vi "Broadcast Sonicator Settings.vi"(8 "error in (no error)":errorcluster, 10 "Message Queues":T5, 11 "Scale Module Config":T1={"GUID"="", "Drop Coords"={"Horizontal"=0, "Vertical"=0}, "Process Name"="", "Queue Name"="", "Settings"={"Cycle Period"=500.0, "Mettler"={"VISA resource name"="", "Simulated?"=FALSE}, "Scale Type"=""}, "Load Count"=0}) -> (0 "error out":errorcluster)   [LabVIEW 2018, in "Sonicator Module.lvlib"]
uses:
  Sonicator Module.lvlib
  Sonicator Message Queues.ctl
  support/Message Queue/Message Cluster.ctl
  Controls/Sonicator Module Config Cluster.ctl
  <vilib>/Utility/miscctls.llb/LVPoint32TypeDef.ctl
  Controls/Sonicator Module Settings Cluster.ctl
  Mettler Toledo/Controls/Settings Cluster.ctl
  support/Message Queue/Enqueue Message (Single).vi
  support/Message Queue/Message Queue.lvlib
  Mettler Toledo/Mettler Toledo.lvlib
panel:
  # "Scale Settings"
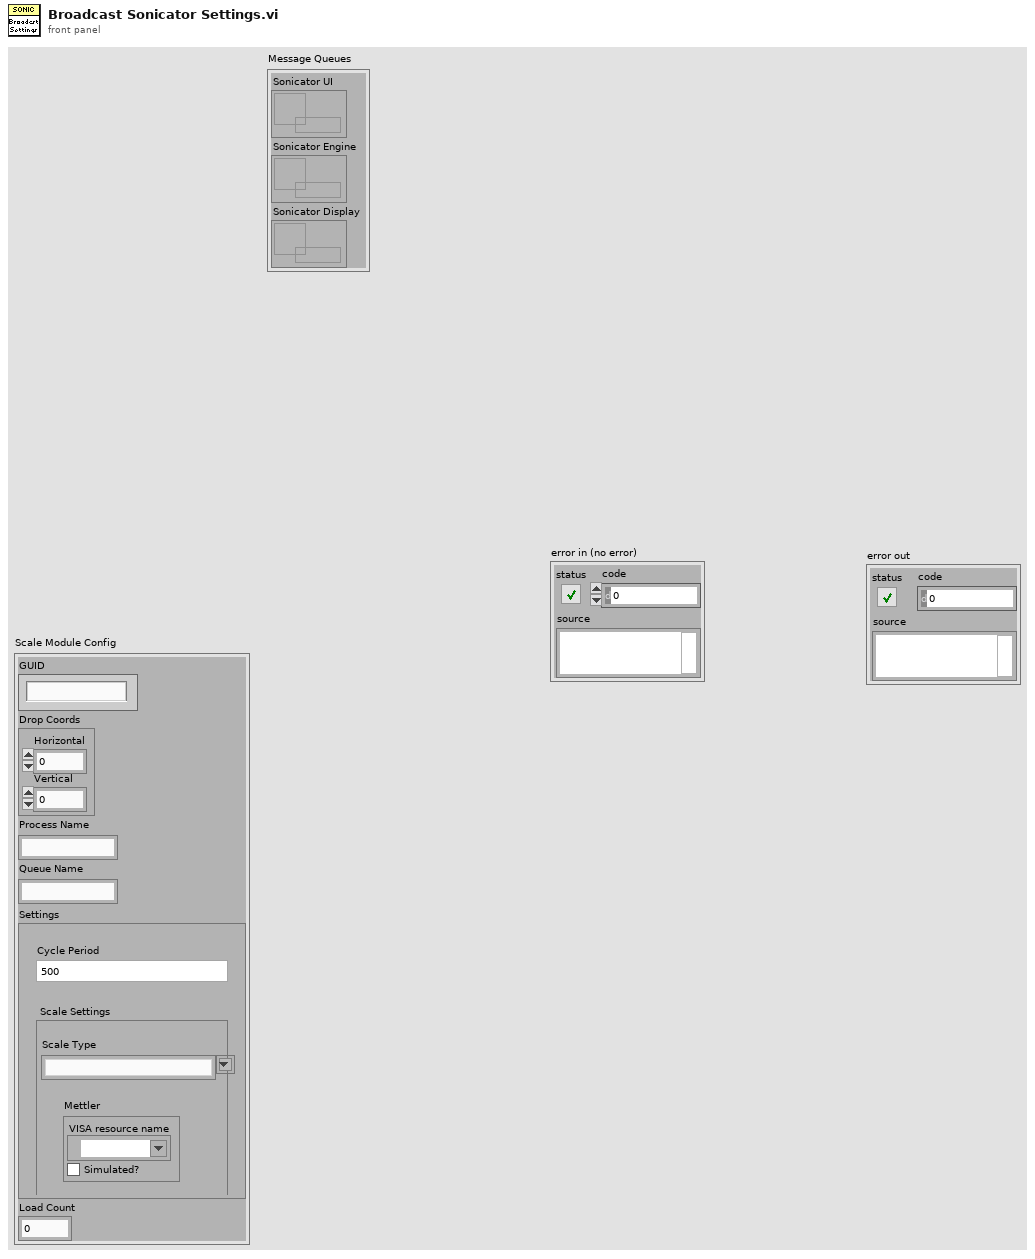
[diagram p1: front panel]
types:
  T1 = typedef "Sonicator Module.lvlib/Sonicator Module Config Cluster.ctl" = cluster{"GUID":string, "Drop Coords":T2, "Process Name":string, "Queue Name":string, "Settings":T3, "Load Count":i32}
  T2 = typedef "LVPoint32TypeDef.ctl" = cluster{"Horizontal":i32, "Vertical":i32}
  T3 = typedef "Sonicator Module.lvlib/Sonicator Module Settings Cluster.ctl" = cluster{"Cycle Period":dbl, "Mettler":T4, "Scale Type":string}
  T4 = typedef "Mettler Toledo.lvlib/Settings Cluster.ctl" = cluster{"VISA resource name":refnum<visa-resource-name>, "Simulated?":bool}
  T5 = typedef "Sonicator Module.lvlib/Sonicator Message Queues.ctl" = cluster{"Sonicator UI":refnum<queue>, "Sonicator Engine":refnum<queue>, "Sonicator Display":refnum<queue>}
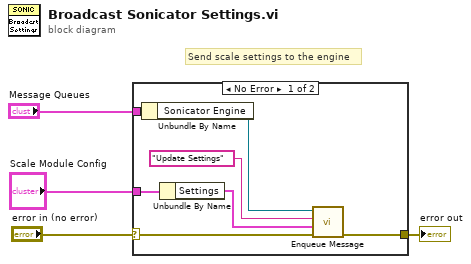
[diagram p0: block diagram]
diagram:
  # "Send scale settings to the engine"
  n1 = case shown="No Error" "error in (no error)" {
    selector: "error in (no error)" -> [w6 w12]
    tunnel: [w5 w12] -> w2
    tunnel: "Scale Module Config" -> [w11 _]
    tunnel: "Message Queues" -> [w10 _]
    frame No Error {
      n2 = Unbundle By Name(w10) -> ("Sonicator Engine"=w9:refnum<queue>)
      n3 = Unbundle By Name(w11) -> ("Settings"=w8:T3)
      n4 = call-poly "Enqueue Message.vi"("error in (no error)"=w6, "Message Data"=w8, "Message"="Update Settings", "Message Queue"=w9) -> ("error out"=w5:errorcluster)  [unwired: 6 in, 1 out]
    }
    frame Error {
    }
  }
  "error out" <- w2
